vi "Pack for gRPC.vi"(8 "error in":errorcluster, 9 "configuration / results":enum16{"Configuration", "Results"}(ring), 10 "data value":variant, 11 "measurement plugin in":refnum<class "Automotive Ethernet Frame Generator.lvclass">) -> (0 "error out":errorcluster, 2 "any":T1, 3 "measurement plugin out":refnum<class "Automotive Ethernet Frame Generator.lvclass">)   [LabVIEW 2025, in "Automotive Ethernet Frame Generator.lvclass"]
uses:
  Automotive Ethernet Frame Generator.lvclass
  Automotive Ethernet Frame Generator.lvclass/Automotive Ethernet Frame Generator.ctl
  C:/Program Files/National Instruments/LabVIEW 2025/vi.lib/Plug-In SDKs/Measurements/Measurement Plugin Service/Measurement Plugin Service.lvclass
  C:/Users/Admin/Documents/jrosartb/hardware-validation/src/labview/auto-eth-frame-generation/Automotive Ethernet Frame Generator/Automotive Ethernet Frame Generator.lvclass
  Measurement Configuration.ctl
  Measurement Results.ctl
  a6012965-5700-4384-8228-972e71b6560c.vi
  2eca732d-dbaa-43bf-a7dd-ede2da65bc1b.vi
  <vilib>/Plug-In SDKs/Measurements/Measurement Plugin Service/Measurement Plugin Service.lvclass
  <vilib>/gRPC/LabVIEW gRPC Library/Shared/Any.ctl
  <vilib>/gRPC/LabVIEW gRPC Library/grpc-lvsupport-release.lvlib
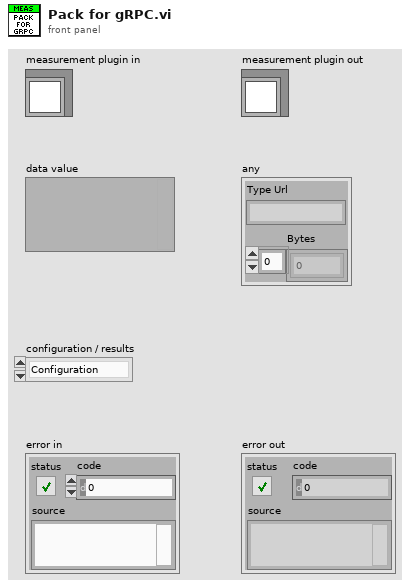
[diagram p1: front panel]
types:
  T1 = typedef "grpc-lvsupport-release.lvlib/Any.ctl" = cluster{"Type Url":string, "Bytes":u8[]}
  T2 = typedef "grpc-lvsupport-release.lvlib/grpcId.ctl" = u64
  T3 = typedef "Automotive Ethernet Frame Generator.lvclass/Measurement Configuration.ctl" = cluster{"INTERFACE NAME STRING":string, "Payload":string, "Protocol Layer 2":cluster{"Has VLAN":bool, "VLAN TAG":cluster{"TPID":u16, "PRIORITY":u8, "DEI":bool, "VID":u16}, "DESTINATION MAC ADDRESS":string, "ETHERTYPE":u16}, "SEND FRAME":bool, "CYCLE?":bool}
  T4 = typedef "Automotive Ethernet Frame Generator.lvclass/Measurement Results.ctl" = cluster{"Transmitting":bool, "RECEIVED PACKETS":i32, "STATUS":string, "OOB gRPC Port":i32}
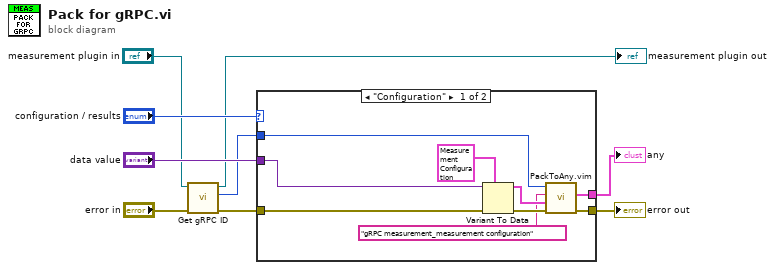
[diagram p0: block diagram]
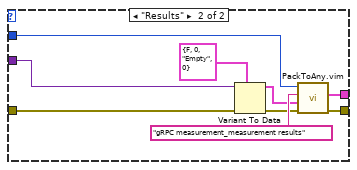
[diagram p2: hidden frame]
diagram:
  n1 = call <vilib>:"Get gRPC ID.vi"("error in"="error in", "measurement plugin service in"="measurement plugin in") -> ("error out"=w4:errorcluster, "gRPC ID"=w1:T2, "measurement plugin service out"=→"measurement plugin out":refnum<class "Automotive Ethernet Frame Generator.lvclass">)  [unwired: 7 in]
  n2 = case shown="\"Configuration\"" "configuration / results" {
    tunnel: w4 -> [w18 w27]
    tunnel: "data value" -> [w17 w26]
    tunnel: w1 -> [w14 w22]
    tunnel: [w16 w24] -> w8
    tunnel: [w15 w23] -> w7
    frame "Configuration" {
      n3 = Variant To Data(error in=w18, type=T3 {"INTERFACE NAME STRING"="Lorem ipsum dolor sit", "Payload"="", "Protocol Layer 2"={"Has VLAN"=FALSE, "VLAN TAG"={"TPID"=0, "PRIORITY"=0, "DEI"=FALSE, "VID"=0}, "DESTINATION MAC ADDRESS"="", "ETHERTYPE"=0}, "SEND FRAME"=TRUE, "CYCLE?"=FALSE} ("measurement configuration"), Variant=w17) -> (data=w13:T3, error out=w12:errorcluster)
      n4 = call "PackToAny.vim"("error in"=w12, "Data To Pack"=w13, "Message Type"="gRPC measurement_measurement configuration", "gRPCid in"=w14) -> ("error out"=w16:errorcluster, "Any"=w15:T1)  [unwired: 5 in, 1 out]
    }
    frame "Results" {
      n5 = Variant To Data(error in=w27, type=T4 {"Transmitting"=FALSE, "RECEIVED PACKETS"=0, "STATUS"="Empty", "OOB gRPC Port"=0} ("Measurement Results"), Variant=w26) -> (data=w20:T4, error out=w19:errorcluster)
      n6 = call "PackToAny.vim"("error in"=w19, "Data To Pack"=w20, "Message Type"="gRPC measurement_measurement results", "gRPCid in"=w22) -> ("error out"=w24:errorcluster, "Any"=w23:T1)  [unwired: 5 in, 1 out]
    }
  }
  "error out" <- w8
  "any" <- w7
